vi "set_speed.vi"(8 "error in (no error)":errorcluster caption="错误输入（无错误）", 10 "speed":i32, 11 "OneMotion 输入":refnum<class "OneMotion.lvclass">) -> (0 "error out":errorcluster caption="错误输出", 3 "OneMotion 输出":refnum<class "OneMotion.lvclass">)   [LabVIEW 2016, in "MotionControl_UFO_3DOF.lvlib" / "OneMotion.lvclass"]
uses:
  <userlib>/MotionControl_UFO_3DOF/OneMotion/OneMotion.lvclass
  <userlib>/MotionControl_UFO_3DOF/OneMotion/OneMotion.lvclass/OneMotion.ctl
  <userlib>/MotionControl_UFO_3DOF/StepMotor/StepMotor.lvclass
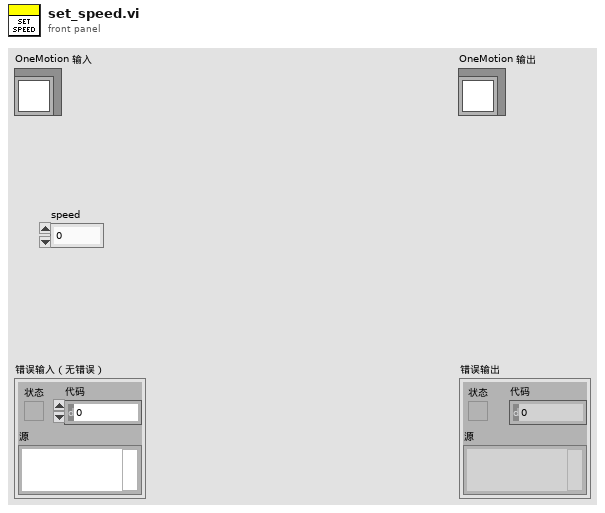
[diagram p1: front panel]
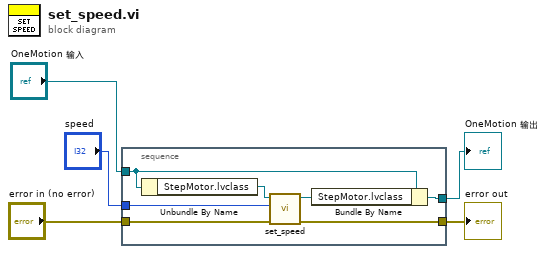
[diagram p0: block diagram]
diagram:
  n1 = stacked-sequence {
    tunnel: [w11] -> w5
    tunnel: [w6] -> w3
    tunnel: "OneMotion 输入" -> [w8]
    tunnel: "speed" -> [w9]
    tunnel: "error in (no error)" -> [w10]
    frame #0 {
      n2 = Unbundle By Name(w8) -> ("StepMotor.lvclass"=w12:refnum<class "StepMotor.lvclass">)
      n3 = call-dynamic "set_speed.vi"("error in (no error)"=w10, "speed"=w9, "StepMotor 输入"=w12) -> ("error out"=w11:errorcluster, "StepMotor 输出"=w7:refnum<class "StepMotor.lvclass">)  [unwired: 7 in]
      n4 = Bundle By Name(cluster=w8, "StepMotor.lvclass"=w7) -> (w6:refnum<class "OneMotion.lvclass">)
    }
  }
  "error out" <- w5
  "OneMotion 输出" <- w3
